vi "Help UI.vi"(8 "error in (no error)":errorcluster) -> (0 "error out":errorcluster)   [LabVIEW 2025, in "Analog Tachometer Process.lvlib" / "Analog Tachometer Process.lvclass"]
uses:
  Analog Tachometer Process.lvclass
panel:
  in  "Tab Control":enum32{"Information", "Figure"}(tab)
  in  "Close Button":bool
  # "The Analog Tachometer Process plugin locates tachometer pulse positions in analog tachometer signals using the number of generated pulses per revolution, the pulse width, and the arrival edge of the tachometer pulse.\n\nParameters\n\nPulse/revolution: specifies the number of pulses the tachometer generates during each revolution. The default is 1.\n\nThreshold: specifies the trigger level that a tachometer pulse must cross to be considered valid. The default is 0.00.\n\nHysteresis: specifies a level above or below the threshold level. Use hysteresis to reduce false triggering that noise in an analog tachometer signal might cause. When the slope is Rising, the analog tachometer signal must fall below threshold minus hysteresis before this plugin detects the next pulse. When the slope is Falling, the analog tachometer signal must rise above threshold plus hysteresis before this plugin detects the next pulse. The default is 0.00.\n\nPulse width: specifies the minimum number of points a valid tachometer pulse must contain. pulse width must be greater than zero. The default is 2.\n\nSlope: specifies the type of edge that indicates the arrival of a tachometer pulse:\n—Rising (default): specifies that a rising edge indicates the arrival of a tachometer pulse.\n—Falling: specifies that a falling edge indicates the arrival of a tachometer pulse.\n\nSelect Channel: this channel specifies the input analog tachometer signal.\n\nOutput Channels\n\nCurrent speed [RPM]: returns the current rotational speed, in revolutions per minute.\nSamples per Revolution: returns the number of samples per revolution."
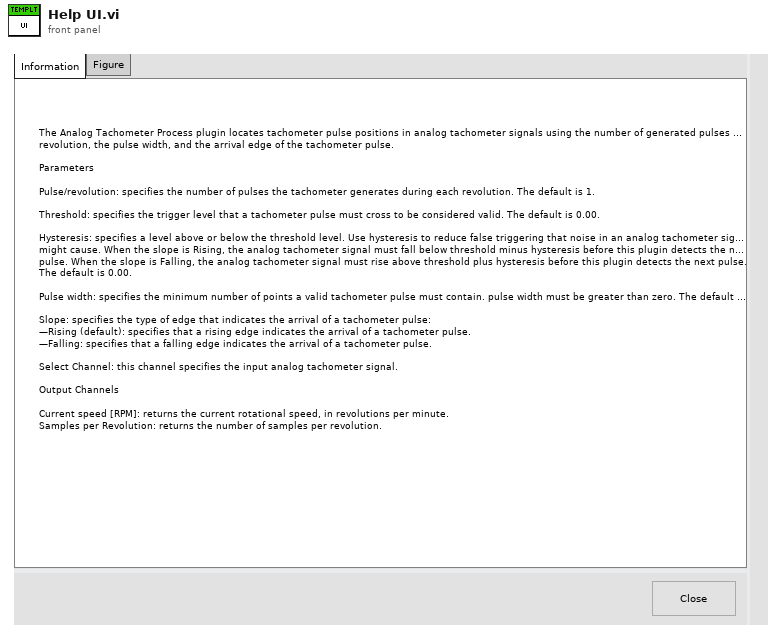
[diagram p1: front panel]
types:
  T1 = enum32{"Invalid", "Standard", "Closed", "Hidden", "Minimized", "Maximized"}
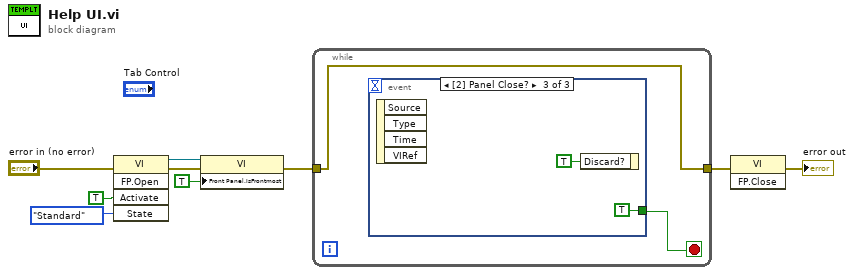
[diagram p0: block diagram]
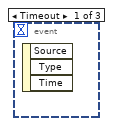
[diagram p2: hidden frame]
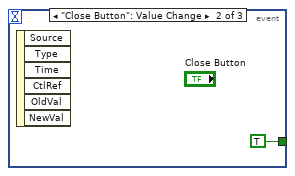
[diagram p3: hidden frame]
diagram:
  n1 = invoke class="VI" method="FP.Open"(error in="error in (no error)", "Activate"=TRUE ("Activate?"), "State"=T1."Standard") -> (reference out=w6:refnum<vi>, error out=w5:errorcluster)  [unwired: 2 in, 3 out]
  n2 = property class="VI"(reference=w6, error in=w5, "Front Panel.IsFrontmost"=TRUE ("Front Panel Window:Is Frontmost")) -> (error out=w4:errorcluster)  [unwired: 1 out]
  n3 = while {
    tunnel: w4 -> [w10]
    tunnel: [w10] -> w3
    stop <- w11 stop-if-true
    n4 = event shown="[2] Panel Close?" {
      selector: _ -> [_ _ _]
      dyn-events: _ -> [_ _ _]
      timeout: _ -> [_ _ _]
      tunnel: [_ TRUE ("Boolean") TRUE ("Boolean")] -> w11
      event Timeout {
        n5 = event-data() -> ()  [unwired: 1 in, 3 out]
      }
      event "Close Button": Value Change {
        n6 = event-data() -> ()  [unwired: 1 in, 6 out]
      }
      event Panel Close? {
        n7 = event-data() -> ()  [unwired: 1 in, 4 out]
        n8 = event-data("Discard?"=TRUE) -> ()  [unwired: 1 in, 1 out]
      }
    }
  }
  n9 = invoke class="VI" method="FP.Close"(error in=w3) -> (error out=→"error out":errorcluster)  [unwired: 2 in, 2 out]
